vi "TDT Synapse Interface.vi"() -> ()   [LabVIEW 2020]
uses:
  Synapse API VIs/SynapseAPI-Mode.ctl
panel:
  out "Block Name":string
  out "Busy":bool
  out "Ready":bool caption="Wait: Initializing hardware..."
  out "Client":bool
  in  "stop":bool
  # "Common Average Referencing"
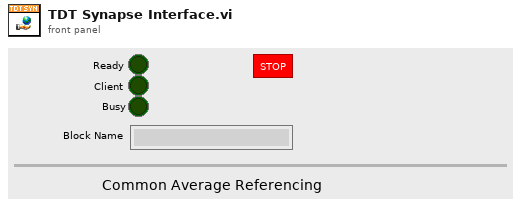
[diagram p1: front panel]
types:
  T1 = typedef "TDTSyn-Settings.ctl" = cluster{"Server IP Address":u32, "TCP Port":u16, "Synapse URL":string, "Tank Root":string}
  T2 = typedef "TDTSyn-State.ctl" = cluster{"TTankX":refnum<k7>, "LastTime":dbl[], "error":errorcluster, "Block Name":string, "Tank Name":string, "NumTicks":i32, "LastTick":dbl[], "LastArtf":dbl, "ChanCount":i32[], "TickSource":i32, "Tank Codes":string[], "waves Tlast":dbl}
  T3 = typedef "SynapseAPI-Mode.ctl" = enum16{"Idle", "Standby", "Preview", "Record"}
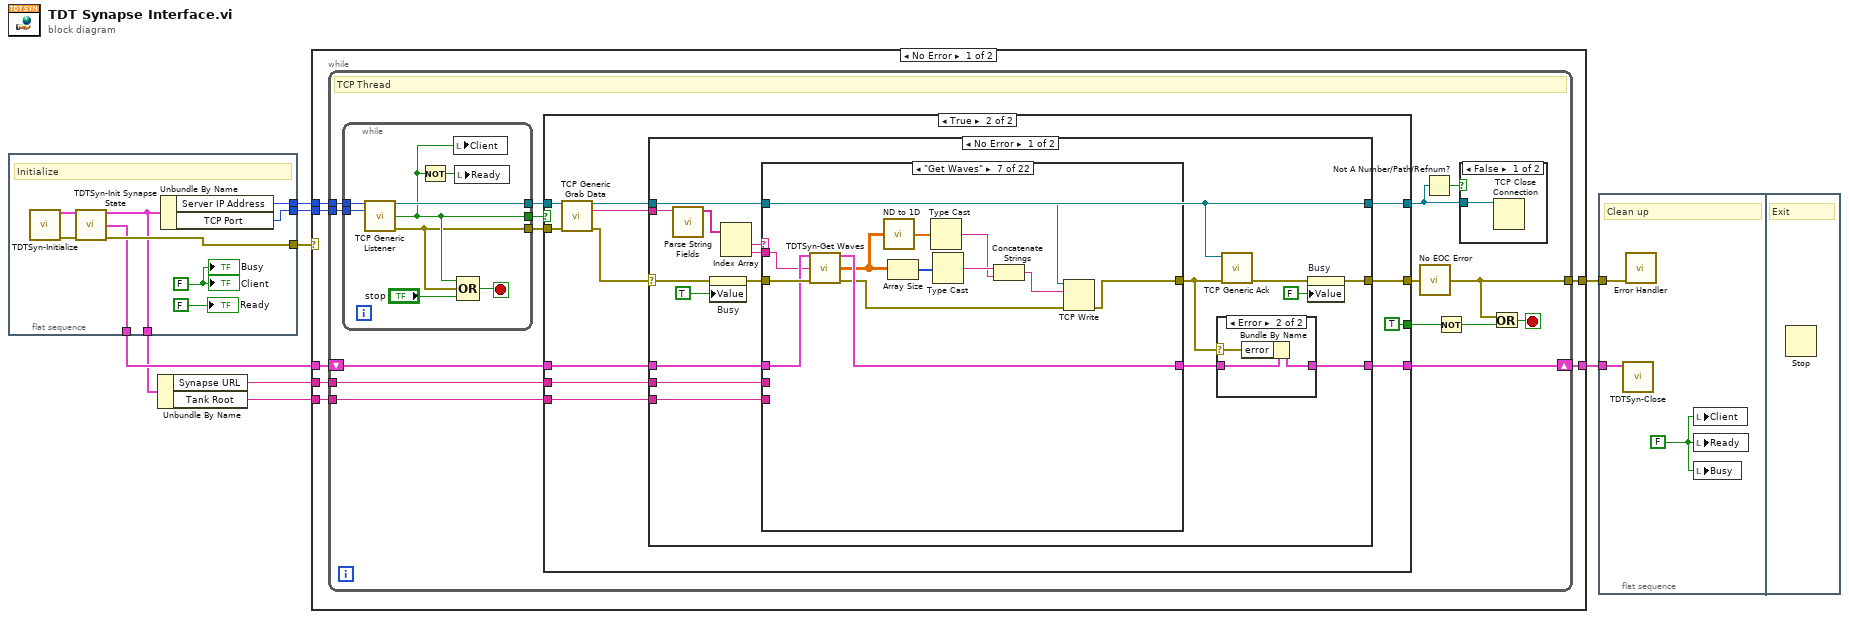
[diagram p0: block diagram]
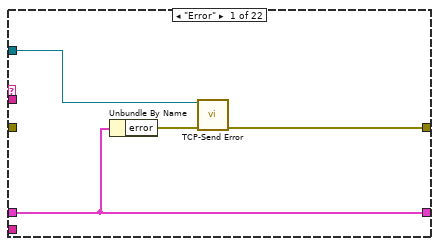
[diagram p5: hidden frame]
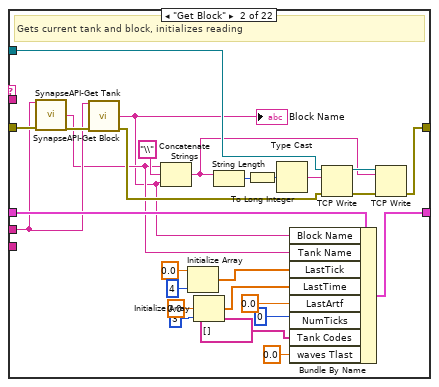
[diagram p6: hidden frame]
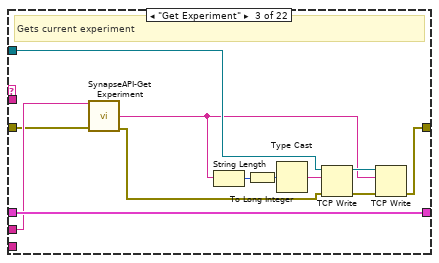
[diagram p7: hidden frame]
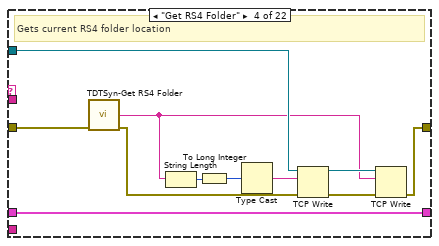
[diagram p8: hidden frame]
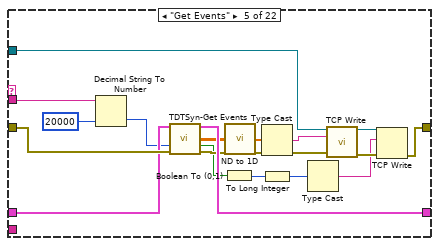
[diagram p9: hidden frame]
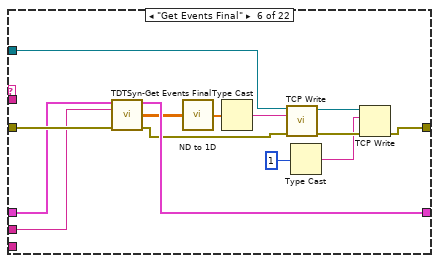
[diagram p10: hidden frame]
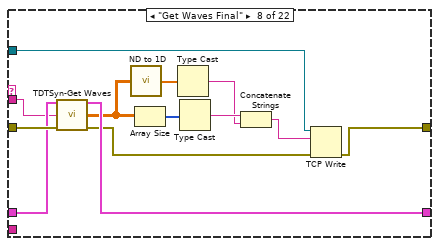
[diagram p11: hidden frame]
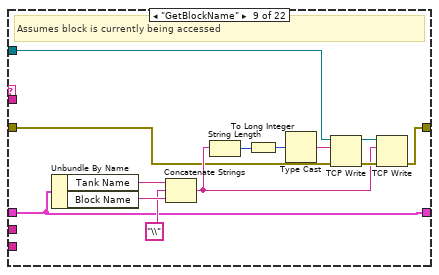
[diagram p12: hidden frame]
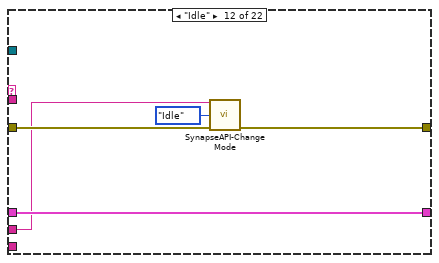
[diagram p15: hidden frame]
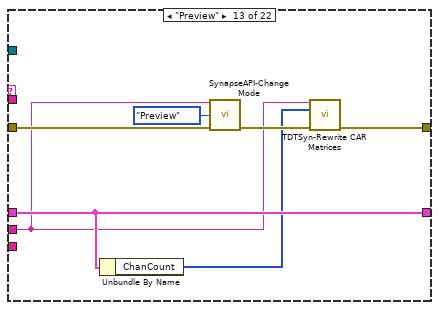
[diagram p16: hidden frame]
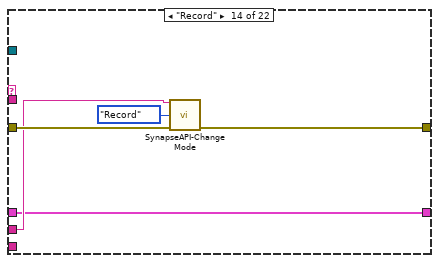
[diagram p17: hidden frame]
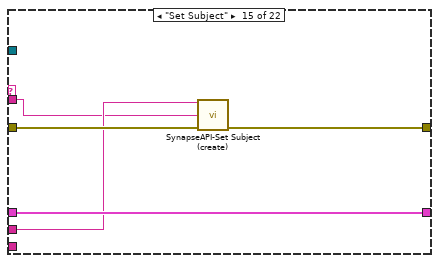
[diagram p18: hidden frame]
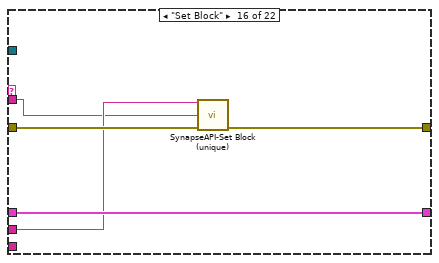
[diagram p19: hidden frame]
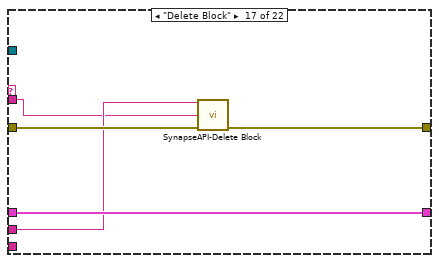
[diagram p20: hidden frame]
diagram:
  n1 = flat-sequence {
    tunnel: [w16] -> w6
    tunnel: [w15] -> w5
    tunnel: [w13] -> w4
    tunnel: [w12] -> w9
    tunnel: [w10] -> w2
    frame #0 {
      w17 = FALSE
      # "Initialize"
      n2 = call "TDTSyn-Initialize.vi"() -> ("Settings"=w11:T1, "error out"=w14:errorcluster)  [unwired: 14 in]
      n3 = call "TDTSyn-Init Synapse State.vi"("Settings"=w11, "error in (no error)"=w14) -> ("Settings (thru)"=w10:T1, "State"=w12:T2, "error out"=w13:errorcluster)  [unwired: 11 in]
      n4 = Unbundle By Name(w10) -> ("Server IP Address"=w16:u32, "TCP Port"=w15:u16)
      "Client" <- w17
      "Ready" <- FALSE
      "Busy" <- w17
    }
  }
  n5 = Unbundle By Name(w2) -> ("Synapse URL"=w8:string, "Tank Root"=w1:string)
  n6 = case shown="No Error" w4 {
    selector: w4 -> [_ w294]
    tunnel: [w25 w294] -> w7
    tunnel: w6 -> [w24 _]
    tunnel: w5 -> [w23 _]
    tunnel: w9 -> [w22 w293]
    tunnel: [w21 w293] -> w3
    tunnel: w8 -> [w20 _]
    tunnel: w1 -> [w19 _]
    frame No Error {
      n7 = while {
        tunnel: [w28] -> w25
        tunnel: w24 -> [w36]
        tunnel: w23 -> [w35]
        shift-right: [w31] -> w21
        shift-left: w22 -> [w32]
        tunnel: w20 -> [w27]
        tunnel: w19 -> [w26]
        stop <- w40 stop-if-true
        # "TCP Thread"
        n8 = while {
          tunnel: [w285] -> w41
          tunnel: [w286] -> w37
          tunnel: w36 -> [w289]
          tunnel: w35 -> [w288]
          tunnel: [w287] -> w34
          stop <- w291 stop-if-true
          n9 = call "TCP Generic Listener.vi"("net address"=w289, "port"=w288) -> ("connection ID"=w287:refnum<k5>, "Connected?"=w286:bool, "error out"=w285:errorcluster)  [unwired: 11 in]
          n10 = Not(x=w286) -> (.not. x?=w290:bool)
          n11 = local write "Client"(w286) -> ()
          n12 = local write "Ready"(w290) -> ()
          n13 = Compound Arithmetic op=OR(w286, w285, "stop") -> (w291:bool)
        }
        n14 = case shown="True" w37 {
          selector: w37 -> [w45 _]
          tunnel: w41 -> [w46 w57]
          tunnel: [w46 w49] -> w33
          tunnel: [w45 TRUE] -> w39
          tunnel: w34 -> [w44 w56]
          tunnel: [w44 w54] -> w29
          tunnel: w32 -> [w43 w52]
          tunnel: [w43 w50] -> w31
          tunnel: w27 -> [_ w48]
          tunnel: w26 -> [_ w47]
          frame False {
          }
          frame True {
            n15 = call "TCP Generic Grab Data.vi"("connection ID"=w56, "error in (no error)"=w57) -> ("connection ID out"=w55:refnum<k5>, "data out"=w58:string, "error out"=w51:errorcluster)  [unwired: 11 in]
            n16 = case shown="No Error" w51 {
              selector: w51 -> [w70 w283]
              tunnel: [w72 w283] -> w49
              tunnel: w58 -> [w64 _]
              tunnel: w55 -> [w68 w284]
              tunnel: [w68 w284] -> w54
              tunnel: w52 -> [w69 w282]
              tunnel: [w65 w282] -> w50
              tunnel: w48 -> [w60 _]
              tunnel: w47 -> [w59 _]
              frame No Error {
                n17 = call "Parse String Fields.vi"("String"=w64) -> ("Fields"=w63:string[])  [unwired: 9 in, 1 out]
                n18 = property on="Busy" class="Bool (strict)"(error in=w70, "Value"=TRUE ("Busy")) -> (error out=w74:errorcluster)  [unwired: 1 in, 1 out]
                n19 = Index Array(array=w63) -> (element #1=w62:string, element #2=w61:string)  [unwired: 2 in]
                n20 = case shown="\"Get Waves\"" w62 {
                  selector: w62 -> [_ _ _ _ _ _ _ _ _ _ _ _ _ _ _ _ _ _ _ _ _ w276]
                  tunnel: w74 -> [_ w97 w112 w124 w151 w165 w178 w191 w192 w206 w208 w210 w219 w224 w229 w234 w239 w247 _ w265 w270 w280]
                  tunnel: [w83 w105 w117 w128 w135 w152 w168 w181 w198 w206 w208 w212 w216 w223 w228 w233 w238 w246 w255 w261 w270 w275] -> w67
                  tunnel: w69 -> [w81 w101 w115 w126 w150 w164 w177 w190 w193 w205 w207 w213 w218 w221 w230 w235 w240 w248 w254 w266 w271 w274]
                  tunnel: [w81 w100 w115 w126 w148 w163 w176 w189 w193 w205 w207 w213 w218 w221 w230 w235 w240 w248 w254 w266 w269 w274] -> w66
                  tunnel: w68 -> [w82 w104 w116 w127 w149 w162 w172 w185 w199 _ _ _ _ _ _ _ _ _ w257 w263 _ _]
                  tunnel: w61 -> [_ _ _ _ w142 _ w174 w187 _ _ _ _ _ _ w226 w231 w236 w243 w252 _ w267 _]
                  tunnel: w60 -> [_ w95 w114 _ _ w157 _ _ _ _ _ w209 w214 w222 w227 w232 w237 w245 _ w260 _ _]
                  tunnel: w59 -> [_ _ _ _ _ _ _ _ _ _ _ _ _ _ _ _ _ w244 _ _ _ _]
                  frame "Error" {
                    n21 = Unbundle By Name(w81) -> ("error"=w80:errorcluster)
                    n22 = call "TCP-Send Error.vi"("connection ID"=w82, "error in (no error)"=w80) -> ("error out"=w83:errorcluster)  [unwired: 13 in]
                  }
                  frame "Get Block" {
                    # "Gets current tank and block, initializes reading"
                    n23 = call "SynapseAPI-Get Tank.vi"("URL"=w95, "error in (no error)"=w97) -> ("tank"=w93:string, "error out"=w96:errorcluster)  [unwired: 12 in]
                    n24 = call "SynapseAPI-Get Block.vi"("URL"=w95, "error in (no error)"=w96) -> ("block"=w92:string, "error out"=w94:errorcluster)  [unwired: 12 in]
                    "Block Name" <- w92
                    n25 = Concatenate Strings(w93, "\\", w92) -> (w99:string)
                    n26 = Initialize Array(0.0 ("element"), 4 ("dimension size")) -> (w89:dbl[])
                    n27 = Initialize Array(0.0 ("element"), 3 ("dimension size")) -> (w85:dbl[])
                    n28 = String Length(string=w99) -> (length=w108:i32)
                    n29 = To Long Integer(number=w108) -> (32bit integer=w107:i32)
                    n30 = Type Cast(x=w107) -> (*(type *) &x=w106:string)  [unwired: 1 in]
                    n31 = Bundle By Name(cluster=w101, "Block Name"=w92, "Tank Name"=w93, "LastTick"=w89, "LastTime"=w85, "LastArtf"=0.0 ("LastTime"), "NumTicks"=0, "Tank Codes"=string[] [], "waves Tlast"=0.0) -> (w100:T2)
                    n32 = TCP Write(connection ID=w104, data in=w106, error in (no error)=w94) -> (connection ID out=w110:refnum<k5>, error out=w109:errorcluster)  [unwired: 1 in, 1 out]
                    n33 = TCP Write(connection ID=w110, data in=w99, error in (no error)=w109) -> (error out=w105:errorcluster)  [unwired: 1 in, 2 out]
                  }
                  frame "Get Experiment" {
                    # "Gets current experiment"
                    n34 = call "SynapseAPI-Get Experiment.vi"("URL"=w114, "error in (no error)"=w112) -> ("experiment"=w111:string, "error out"=w113:errorcluster)  [unwired: 12 in]
                    n35 = String Length(string=w111) -> (length=w120:i32)
                    n36 = To Long Integer(number=w120) -> (32bit integer=w119:i32)
                    n37 = Type Cast(x=w119) -> (*(type *) &x=w118:string)  [unwired: 1 in]
                    n38 = TCP Write(connection ID=w116, data in=w118, error in (no error)=w113) -> (connection ID out=w122:refnum<k5>, error out=w121:errorcluster)  [unwired: 1 in, 1 out]
                    n39 = TCP Write(connection ID=w122, data in=w111, error in (no error)=w121) -> (error out=w117:errorcluster)  [unwired: 1 in, 2 out]
                  }
                  frame "Get RS4 Folder" {
                    # "Gets current RS4 folder location"
                    n40 = call "TDTSyn-Get RS4 Folder.vi"("error in"=w124) -> ("folder"=w123:string, "error out"=w125:errorcluster)  [unwired: 13 in]
                    n41 = String Length(string=w123) -> (length=w131:i32)
                    n42 = To Long Integer(number=w131) -> (32bit integer=w130:i32)
                    n43 = Type Cast(x=w130) -> (*(type *) &x=w129:string)  [unwired: 1 in]
                    n44 = TCP Write(connection ID=w127, data in=w129, error in (no error)=w125) -> (connection ID out=w133:refnum<k5>, error out=w132:errorcluster)  [unwired: 1 in, 1 out]
                    n45 = TCP Write(connection ID=w133, data in=w123, error in (no error)=w132) -> (error out=w128:errorcluster)  [unwired: 1 in, 2 out]
                  }
                  frame "Get Events" {
                    n46 = Decimal String To Number(string=w142, default (0L)=20000 ("default (0 I32)")) -> (number=w141:i32)  [unwired: 1 in, 1 out]
                    n47 = call "TDTSyn-Get Events.vi"("State In"=w150, "Max Read"=w141, "error in (no error)"=w151) -> ("State Out"=w148:T2, "Events"=w145:dbl[][], "backlog"=w138:bool, "error out"=w147:errorcluster)  [unwired: 9 in]
                    n48 = Boolean To (0,1)(Boolean=w138) -> (0, 1=w137:i16)
                    n49 = call "ND to 1D.vi"("ND Array"=w145) -> ("1D Array"=w144:dbl[])
                    n50 = Type Cast(x=w144) -> (*(type *) &x=w146:string)  [unwired: 1 in]
                    n51 = To Long Integer(number=w137) -> (32bit integer=w134:i32)
                    n52 = Type Cast(x=w134) -> (*(type *) &x=w136:string)  [unwired: 1 in]
                    n53 = call "TCP Write.vi"("connection ID"=w149, "data string"=w146, "error in (no error)"=w147) -> ("connection ID out"=w140:refnum<k5>, "error out"=w139:errorcluster)  [unwired: 10 in, 1 out]
                    n54 = TCP Write(connection ID=w140, data in=w136, error in (no error)=w139) -> (error out=w135:errorcluster)  [unwired: 1 in, 2 out]
                  }
                  frame "Get Events Final" {
                    n55 = call "TDTSyn-Get Events Final.vi"("State"=w164, "URL"=w157, "error in (no error)"=w165) -> ("Data out"=w163:T2, "Events"=w159:dbl[][], "error out"=w161:errorcluster)  [unwired: 8 in, 2 out]
                    n56 = call "ND to 1D.vi"("ND Array"=w159) -> ("1D Array"=w158:dbl[])
                    n57 = Type Cast(x=w158) -> (*(type *) &x=w160:string)  [unwired: 1 in]
                    n58 = call "TCP Write.vi"("connection ID"=w162, "data string"=w160, "error in (no error)"=w161) -> ("connection ID out"=w154:refnum<k5>, "error out"=w155:errorcluster)  [unwired: 10 in, 1 out]
                    n59 = Type Cast(x=1) -> (*(type *) &x=w153:string)  [unwired: 1 in]
                    n60 = TCP Write(connection ID=w154, data in=w153, error in (no error)=w155) -> (error out=w152:errorcluster)  [unwired: 1 in, 2 out]
                  }
                  frame "Get Waves" {
                    n61 = call "TDTSyn-Get Waves.vi"("State In"=w177, "codes"=w174, "error in (no error)"=w178) -> ("State Out"=w176:T2, "Waves"=w173:dbl[][], "error out"=w171:errorcluster)  [unwired: 10 in]
                    n62 = call "ND to 1D.vi"("ND Array"=w173) -> ("1D Array"=w175:dbl[])
                    n63 = Array Size(array=w173) -> (size(s)=w170:i32[])
                    n64 = Type Cast(x=w175) -> (*(type *) &x=w166:string)  [unwired: 1 in]
                    n65 = Type Cast(x=w170) -> (*(type *) &x=w169:string)  [unwired: 1 in]
                    n66 = Concatenate Strings(w169, w166) -> (w167:string)
                    n67 = TCP Write(connection ID=w172, data in=w167, error in (no error)=w171) -> (error out=w168:errorcluster)  [unwired: 1 in, 2 out]
                  }
                  frame "Get Waves Final" {
                    n68 = call "TDTSyn-Get Waves.vi"("State In"=w190, "codes"=w187, "error in (no error)"=w191) -> ("State Out"=w189:T2, "Waves"=w186:dbl[][], "error out"=w184:errorcluster)  [unwired: 10 in]
                    n69 = call "ND to 1D.vi"("ND Array"=w186) -> ("1D Array"=w188:dbl[])
                    n70 = Array Size(array=w186) -> (size(s)=w183:i32[])
                    n71 = Type Cast(x=w188) -> (*(type *) &x=w179:string)  [unwired: 1 in]
                    n72 = Type Cast(x=w183) -> (*(type *) &x=w182:string)  [unwired: 1 in]
                    n73 = Concatenate Strings(w182, w179) -> (w180:string)
                    n74 = TCP Write(connection ID=w185, data in=w180, error in (no error)=w184) -> (error out=w181:errorcluster)  [unwired: 1 in, 2 out]
                  }
                  frame "GetBlockName" {
                    # "Assumes block is currently being accessed"
                    n75 = Unbundle By Name(w193) -> ("Tank Name"=w196:string, "Block Name"=w195:string)
                    n76 = Concatenate Strings(w196, "\\", w195) -> (w197:string)
                    n77 = String Length(string=w197) -> (length=w202:i32)
                    n78 = To Long Integer(number=w202) -> (32bit integer=w201:i32)
                    n79 = Type Cast(x=w201) -> (*(type *) &x=w200:string)  [unwired: 1 in]
                    n80 = TCP Write(connection ID=w199, data in=w200, error in (no error)=w192) -> (connection ID out=w204:refnum<k5>, error out=w203:errorcluster)  [unwired: 1 in, 1 out]
                    n81 = TCP Write(connection ID=w204, data in=w197, error in (no error)=w203) -> (error out=w198:errorcluster)  [unwired: 1 in, 2 out]
                  }
                  frame "NOOP" {
                    # "do nothing"
                  }
                  frame "Ping" {
                  }
                  frame "Idle" {
                    n82 = call "SynapseAPI-Change Mode.vi"("URL"=w209, "mode"=SynapseAPI-Mode."Idle", "error in (no error)"=w210) -> ("error out"=w212:errorcluster)  [unwired: 12 in]
                  }
                  frame "Preview" {
                    n83 = Unbundle By Name(w218) -> ("ChanCount"=w215:i32[])
                    n84 = call "SynapseAPI-Change Mode.vi"("URL"=w214, "mode"=SynapseAPI-Mode."Preview", "error in (no error)"=w219) -> ("error out"=w217:errorcluster)  [unwired: 12 in]
                    n85 = call "TDTSyn-Rewrite CAR Matrices.vi"("URL"=w214, "ChanCount"=w215, "error in (no error)"=w217) -> ("error out"=w216:errorcluster)  [unwired: 12 in]
                  }
                  frame "Record" {
                    n86 = call "SynapseAPI-Change Mode.vi"("URL"=w222, "mode"=SynapseAPI-Mode."Record", "error in (no error)"=w224) -> ("error out"=w223:errorcluster)  [unwired: 12 in]
                  }
                  frame "Set Subject" {
                    n87 = call "SynapseAPI-Set Subject (create).vi"("URL"=w227, "subject"=w226, "error in (no error)"=w229) -> ("error out"=w228:errorcluster)  [unwired: 12 in]
                  }
                  frame "Set Block" {
                    n88 = call "SynapseAPI-Set Block (unique).vi"("URL"=w232, "block"=w231, "error in (no error)"=w234) -> ("error out"=w233:errorcluster)  [unwired: 12 in]
                  }
                  frame "Delete Block" {
                    n89 = call "SynapseAPI-Delete Block.vi"("URL"=w237, "block"=w236, "error in (no error)"=w239) -> ("error out"=w238:errorcluster)  [unwired: 12 in]
                  }
                  frame "Set Tank" {
                    n90 = Concatenate Strings(w244, "\\" ("element"), w243) -> (w241:string)
                    n91 = call "SynapseAPI-Set Tank (create).vi"("URL"=w245, "tank"=w241, "error in (no error)"=w247) -> ("error out"=w246:errorcluster)  [unwired: 12 in]
                  }
                  frame "SpeedTest" {
                    n92 = Decimal String To Number(string=w252, default (0L)=1 ("default (0 I32)")) -> (number=w250:i32)  [unwired: 1 in, 1 out]
                    n93 = Initialize Array(3.7, w250) -> (w251:dbl[])
                    n94 = Type Cast(x=w251) -> (*(type *) &x=w256:string)  [unwired: 1 in]
                    n95 = call "TCP Write.vi"("connection ID"=w257, "data string"=w256) -> ("error out"=w255:errorcluster)  [unwired: 11 in, 2 out]
                  }
                  frame "Status" {
                    n96 = call "SynapseAPI-Get Mode.vi"("URL"=w260, "error in (no error)"=w265) -> ("mode"=w262:T3, "error out"=w264:errorcluster)  [unwired: 12 in]
                    n97 = To Long Integer(number=w262) -> (32bit integer=w258:i32)
                    n98 = Type Cast(x=w258) -> (*(type *) &x=w259:string)  [unwired: 1 in]
                    n99 = TCP Write(connection ID=w263, data in=w259, error in (no error)=w264) -> (error out=w261:errorcluster)  [unwired: 1 in, 2 out]
                  }
                  frame "Tick Source" {
                    n100 = case shown="\"Tosca\"" w267 {
                      tunnel: [0 3] -> w268
                      frame "", Default {
                      }
                      frame "Tosca" {
                      }
                    }
                    n101 = Bundle By Name(cluster=w271, "TickSource"=w268) -> (w269:T2)
                  }
                  frame Default {
                    w279 = 1 items=["No error", "Argument error", "Memory is full", "Out of zone", "End of file", "File already open", "Generic file I/O error", "File not found", "File permission error", "Disk is full", "Duplicate path", "Too many files open", "System feature not enabled", "Resource file not found", "Cannot add resource", "Resource not found", "Image not found", "Image memory error", "Pen does not exist", "Config type invalid", "Config token not found", "Config parse error", "Config memory error", "Bad external code format", "Bad external code offset", "External code not present", "Null window", "Destroy window error", "Null menu", "Print aborted", "Bad print record", "Print driver error", "Windows error during printing", "Memory error during printing", "Print dialog error", "Generic print error", "Invalid device refnum", "Device not found", "Device parameter error", "Device unit error", "Cannot open device", "Device call aborted", "Generic error", "Cancelled by user", "Object ID too low", "Object ID too high", "Object not in heap", "Unknown heap", "Unknown object (invalid DefProc)", "Unknown object (DefProc not in table)", "Message out of range", "Invalid (null) method", "Unknown message", "Manager call not supported", "Bad address", "Network operation in progress", "Network operation timed out", "Connection is busy", "Network attribute not supported", "Network error", "Address in use", "System out of memory", "Connection aborted", "Connection refused", "Not connected", "Already connected", "Connection closed", "Initialization error (interapplication manager)", "Bad occurrence", "Wait on unbound occurrence handler", "Occurrence queue overflow", "Datalog type conflict", "Unused", "Unrecognized type (interapplication manager)", "Memory corrupt", "Failed to make temporary DLL", "Old CIN version", "Drag socket not found", "Failed to load drop-object", "Failed to register OLE object", "Failed to release OLE object", "Format specifier type mismatch", "Unknown format specifier", "Too few format specifiers", "Too many format specifiers", "Scan failed", "Newer CIN version", "Error converting to variant", "Runtime menu error", "Password tampered", "Variant attribute not found", "Incompatible variant data type", "Event data is not available", "Event Store is not present", "Occurrence is not found", "Event Queue is not created", "Event info is not available", "Refnum passed is NULL", "Error retrieving Class GUID", "Error retrieving CoClass GUID", "Error retrieving TypeLib GUID.", "Bad built application magic bytes.", "Specific driver is different from the specific driver associated with the Logical Name.", "There is no session opened to the class driver.", "Max Error", "MAX - Error with config objects", "MAX - Error loading configuration", "MAX - Group not supported"]
                    n102 = Format Into String(format string="Unrecognized TCP command '%s'", w276) -> (resulting string=w281:string)  [unwired: 2 in, 1 out]
                    n103 = Bundle By Name(cluster=w280, "code"=w279, "status"=TRUE, "source"=w281) -> (w275:errorcluster)
                  }
                }
                n104 = case shown="Error" w67 {
                  selector: w67 -> [_ w77]
                  tunnel: w66 -> [w76 w79]
                  tunnel: [w76 w78] -> w65
                  frame No Error {
                  }
                  frame Error {
                    n105 = Bundle By Name(cluster=w79, "error"=w77) -> (w78:T2)
                  }
                }
                n106 = call "TCP Generic Ack.vi"("connection ID"=w68, "error in (no error)"=w67) -> ("error out"=w73:errorcluster)  [unwired: 7 in, 1 out]
                n107 = property on="Busy" class="Bool (strict)"(error in=w73, "Value"=FALSE ("Busy")) -> (error out=w72:errorcluster)  [unwired: 1 in, 1 out]
              }
              frame Error {
              }
            }
          }
        }
        n108 = call "No EOC Error.vi"("error in"=w33) -> ("error out"=w28:errorcluster)  [unwired: 4 in]
        n109 = Not A Number/Path/Refnum?(number/path/refnum=w29) -> (NaN/Path/Refnum?=w30:bool)
        n110 = Not(x=w39) -> (.not. x?=w38:bool)
        n111 = case shown="False" w30 {
          tunnel: w29 -> [w42 _]
          frame False {
            n112 = TCP Close Connection(connection ID=w42) -> ()  [unwired: 2 in, 2 out]
          }
          frame True {
          }
        }
        n113 = Or(x=w28, y=w38) -> (x .or. y?=w40:bool)
      }
    }
    frame Error {
    }
  }
  n114 = flat-sequence {
    tunnel: w7 -> [w296]
    tunnel: w3 -> [w295]
    frame #0 {
      w297 = FALSE
      # "Clean up"
      n115 = call "TDTSyn-Close.vi"("State in"=w295) -> ()  [unwired: 13 in, 2 out]
      n116 = call "Error Handler.vi"("error in (no error)"=w296) -> ()  [unwired: 13 in, 2 out]
      n117 = local write "Client"(w297) -> ()
      n118 = local write "Ready"(w297) -> ()
      n119 = local write "Busy"(w297) -> ()
    }
    frame #1 {
      # "Exit"
      n120 = Stop() -> ()  [unwired: 1 in]
    }
  }
